vi "Configure OSC Limit Short.vi"(7 "Mode":T2 items=["OSC"], 8 "error in (no error)":errorcluster, 9 "Limit Short":u32 max=5 step=1, 10 "Step":T1=1 min=1 max=99 step=1, 11 "VISA resource name":refnum<visa-resource-name>) -> (0 "error out":errorcluster, 3 "VISA resource name out":refnum<visa-resource-name>)   [LabVIEW 2025]
uses:
  <instrlib>/Chroma 19052/Public/Utility/Type Def/OSC mode--ring.ctl
  <instrlib>/Chroma 19052/Public/Utility/Type Def/steps--numeric.ctl
  <instrlib>/Chroma 19052/Chroma 19052.lvlib
panel:
  # "Configure OSC Limit Short"
  # "0,1...5"
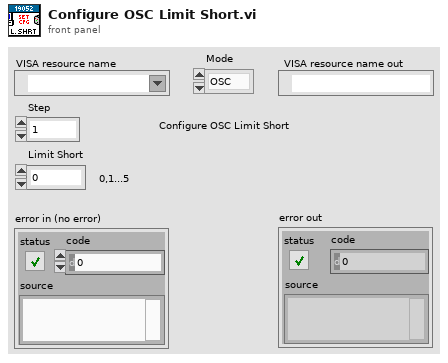
[diagram p1: front panel]
types:
  T1 = typedef "Chroma 19052.lvlib/steps--numeric.ctl" = u8
  T2 = typedef "Chroma 19052.lvlib/OSC mode--ring.ctl" = i32
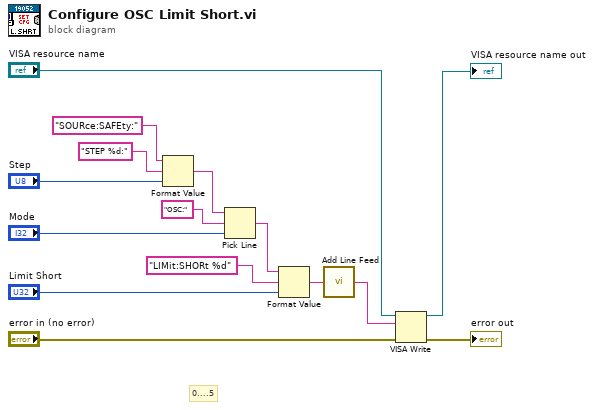
[diagram p0: block diagram]
diagram:
  # "0....5"
  n1 = Format Value(string ("")="SOURce:SAFEty:", format string="STEP %d:", value (0)="Step") -> (output string=w10:string)
  n2 = Pick Line(string ("")=w10, multi-line string="OSC:", line index="Mode") -> (output string=w8:string)
  n3 = Format Value(string ("")=w8, format string="LIMit:SHORt %d", value (0)="Limit Short") -> (output string=w6:string)
  n4 = call <instrlib>:"Add Line Feed.vi"("Command string"=w6) -> ("Concatenated string"=w5:string)  [unwired: 4 in]
  n5 = VISA Write(VISA resource name="VISA resource name", write buffer=w5, error in (no error)="error in (no error)") -> (VISA resource name out=→"VISA resource name out":refnum<visa-resource-name>, error out=→"error out":errorcluster)  [unwired: 1 out]
